vi "SubVI_ResAcc2.vi"() -> ()   [LabVIEW 2013]
uses:
  <vilib>/DAQmx/read.llb/DAQmx Read.vi
  <vilib>/DAQmx/read.llb/DAQmx Read (Analog 1D Wfm NChan NSamp).vi
  <vilib>/DAQmx/create/channels.llb/DAQmx Create Channel (TEDS-AI-Voltage-Basic).vi
  <vilib>/DAQmx/create/channels.llb/DAQmx Create Channel (AI-Voltage-Basic).vi
  <vilib>/DAQmx/configure/timing.llb/DAQmx Timing (Sample Clock).vi
  <vilib>/DAQmx/configure/trigger.llb/DAQmx Trigger.vi
  <vilib>/DAQmx/configure/trigger.llb/DAQmx Start Trigger (Digital Edge).vi
  <vilib>/DAQmx/miscellaneous.llb/DAQmx Fill In Error Info.vi
panel:
  out "task out":refnum<k21> caption="태스크 출력"
  out "error out":errorcluster caption="에러 출력"
  in  "error in":errorcluster caption="에러 입력"
  in  "timeout (s)":dbl=10.0 caption="타임아웃(초)" format="%0.2f"
  out "data":dynamicdata(graph) caption="데이터"
  in  "stop (T)":bool=TRUE caption="정지(T)"
  in  "디바이스 이름":tag="cDAQ1Mod1"
  in  "속도":dbl=100000.0
  in  "샘플 개수":i32=2000
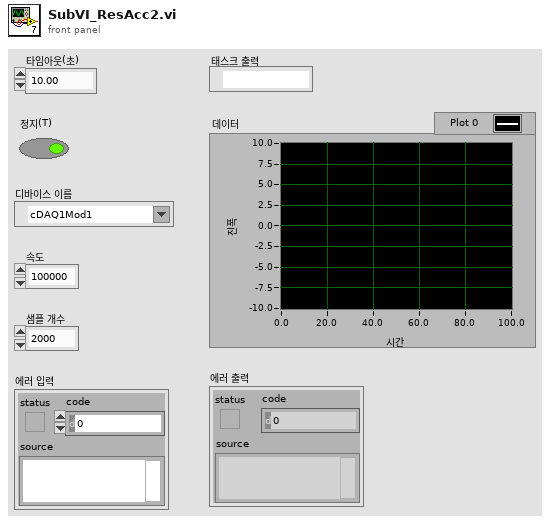
[diagram p1: front panel]
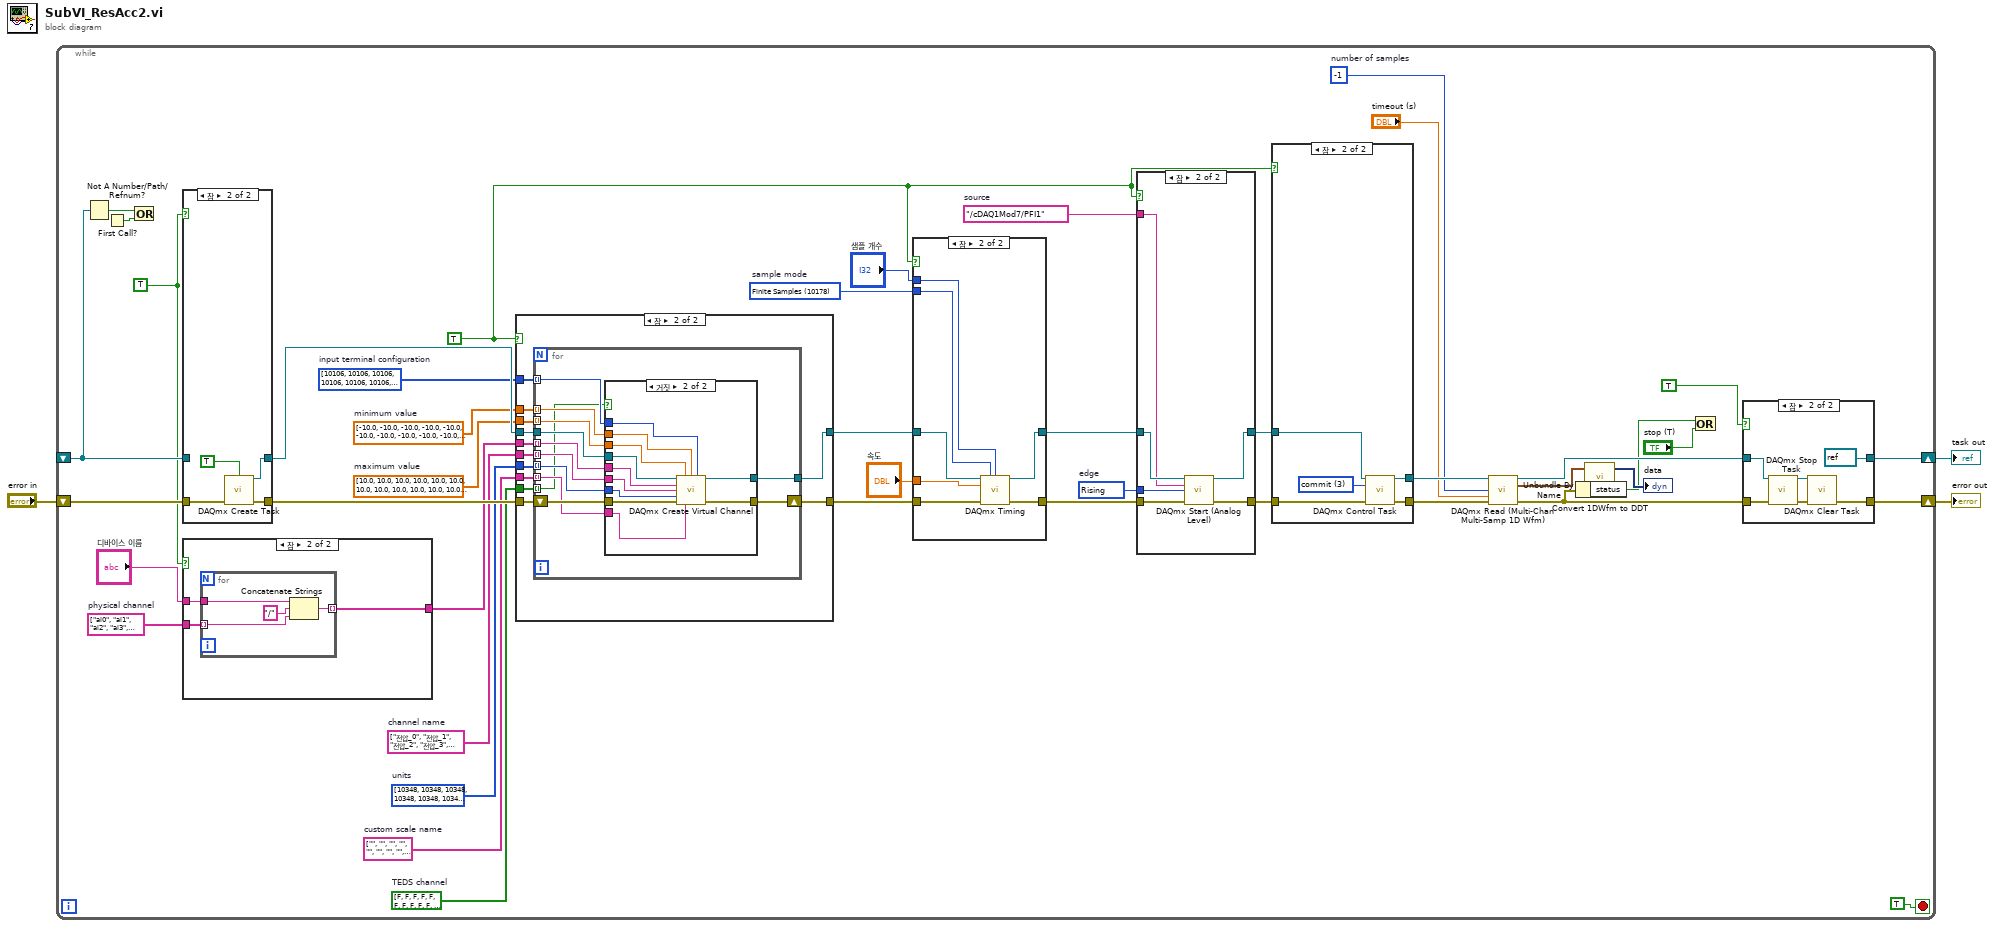
[diagram p0: block diagram]
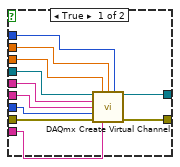
[diagram p7: hidden frame]
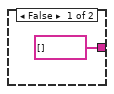
[diagram p8: hidden frame]
diagram:
  n1 = while {
    shift-right: [w12] -> w1
    shift-left: _ -> [w43]
    shift-right: [w10] -> w2
    shift-left: "error in" -> [w44]
    stop <- TRUE stop-if-true
    w5 = TRUE
    w6 = TRUE
    w16 = -1  # number of samples
    w21 = 10280 items=["Rising"=10280, "Falling"=10171]  # edge
    w22 = "/cDAQ1Mod7/PFI1"  # source
    w25 = 10178 items=["Finite Samples"=10178, "Continuous Samples"=10123, "Hardware Timed Single Point"=12522]  # sample mode
    w30 = bool[] [FALSE, FALSE, FALSE, FALSE, FALSE, FALSE, FALSE, FALSE, FALSE, FALSE, FALSE, FALSE, FALSE, FALSE, FALSE, FALSE]  # TEDS channel
    w31 = string[] ["", "", "", "", "", "", "", "", "", "", "", "", "", "", "", ""]  # custom scale name
    w32 = i32[] [10348, 10348, 10348, 10348, 10348, 10348, 10348, 10348, 10348, 10348, 10348, 10348, 10348, 10348, 10348, 10348] items=["Volts"=10348, "From TEDS"=12516, "From Custom Scale"=10065]  # units
    w33 = string[] ["전압_0", "전압_1", "전압_2", "전압_3", "전압_4", "전압_5", "전압_6", "전압_7", "전압_8", "전압_9", "전압_10", "전압_11", "전압_12", "전압_13", "전압_14", "전압_15"]  # channel name
    w35 = dbl[] [10.0, 10.0, 10.0, 10.0, 10.0, 10.0, 10.0, 10.0, 10.0, 10.0, 10.0, 10.0, 10.0, 10.0, 10.0, 10.0]  # maximum value
    w36 = dbl[] [-10.0, -10.0, -10.0, -10.0, -10.0, -10.0, -10.0, -10.0, -10.0, -10.0, -10.0, -10.0, -10.0, -10.0, -10.0, -10.0]  # minimum value
    w37 = i32[] [10106, 10106, 10106, 10106, 10106, 10106, 10106, 10106, 10106, 10106, 10106, 10106, 10106, 10106, 10106, 10106] items=["default"=-1, "RSE"=10083, "NRSE"=10078, "Differential"=10106, "Pseudodifferential"=12529]  # input terminal configuration
    w40 = string[] ["ai0", "ai1", "ai2", "ai3", "ai4", "ai5", "ai6", "ai7", "ai8", "ai9", "ai10", "ai11", "ai12", "ai13", "ai14", "ai15"]  # physical channel
    n2 = Not A Number/Path/Refnum?(number/path/refnum=w43) -> (NaN/Path/Refnum?=w42:bool)
    n3 = First Call?() -> (First Call?: T/F=w45:bool)
    n4 = Or(x=w42, y=w45) -> ()  [unwired: 1 out]
    n5 = case "케이스 구조" shown="참" w5 {
      tunnel: [w136 w140] -> w39
      tunnel: w43 -> [w136 _]
      tunnel: [w135 w139] -> w38
      tunnel: w44 -> [w135 w137]
      frame False {
      }
      frame True {
        n6 = call <vilib>:"DAQmx Create Task.vi"("auto cleanup"=TRUE, "error in"=w137) -> ("task out"=w140:refnum<k21>, "error out"=w139:errorcluster)  [unwired: 12 in]
      }
    }
    n7 = case "케이스 구조" shown="참" w5 {
      tunnel: [string[] [] w130] -> w34
      tunnel: "디바이스 이름" -> [_ w129]
      tunnel: w40 -> [_ w128]
      frame False {
      }
      frame True {
        n8 = for "For 루프" {
          tunnel: [w134] -> w130 mode=indexing
          tunnel: w129 -> [w133]
          tunnel: w128 -> [w131] mode=indexing
          n9 = Concatenate Strings(w133, "/" ("string"), w131) -> (w134:string)
        }
      }
    }
    n10 = case "케이스 구조" shown="참" w6 {
      tunnel: [w80 w90] -> w29
      tunnel: w39 -> [w80 w92]
      tunnel: [w79 w89] -> w28
      tunnel: w38 -> [w79 w91]
      tunnel: w37 -> [_ w88]
      tunnel: w36 -> [_ w87]
      tunnel: w35 -> [_ w86]
      tunnel: w34 -> [_ w85]
      tunnel: w33 -> [_ w84]
      tunnel: w32 -> [_ w83]
      tunnel: w31 -> [_ w82]
      tunnel: w30 -> [_ w81]
      frame False {
      }
      frame True {
        n11 = for "For 루프" {
          tunnel: w92 -> [w104]
          tunnel: [w102] -> w90
          tunnel: w88 -> [w100] mode=indexing
          tunnel: w87 -> [w99] mode=indexing
          tunnel: w86 -> [w98] mode=indexing
          tunnel: w85 -> [w97] mode=indexing
          tunnel: w84 -> [w96] mode=indexing
          tunnel: w83 -> [w95] mode=indexing
          tunnel: w82 -> [w94] mode=indexing
          shift-right: [w101] -> w89
          shift-left: w91 -> [w103]
          tunnel: w81 -> [w93] mode=indexing
          n12 = case "케이스 구조" shown="거짓" w93 {
            tunnel: w104 -> [w115 w126]
            tunnel: w103 -> [w114 w125]
            tunnel: [w113 w124] -> w102
            tunnel: [w112 w123] -> w101
            tunnel: w100 -> [w111 w122]
            tunnel: w99 -> [w110 w121]
            tunnel: w98 -> [w109 w120]
            tunnel: w97 -> [w108 w119]
            tunnel: w96 -> [w107 w118]
            tunnel: w95 -> [w106 w117]
            tunnel: w94 -> [w105 w116]
            frame True {
              n13 = call-poly <vilib>:"DAQmx Create Virtual Channel.vi"("task in"=w115, "maximum value"=w109, "minimum value"=w110, "input terminal configuration"=w111, "physical channels"=w108, "name to assign"=w107, "units"=w106, "error in"=w114, "custom scale name"=w105) -> ("task out"=w113:refnum<k21>, "error out"=w112:errorcluster)  [unwired: 5 in]
            }
            frame False {
              n14 = call-poly <vilib>:"DAQmx Create Virtual Channel.vi"("task in"=w126, "maximum value"=w120, "minimum value"=w121, "input terminal configuration"=w122, "physical channels"=w119, "name to assign"=w118, "units"=w117, "error in"=w125, "custom scale name"=w116) -> ("task out"=w124:refnum<k21>, "error out"=w123:errorcluster)  [unwired: 5 in]
            }
          }
        }
      }
    }
    n15 = case "케이스 구조" shown="참" w6 {
      tunnel: [w71 w73] -> w24
      tunnel: w29 -> [w71 w76]
      tunnel: [w70 w72] -> w23
      tunnel: w28 -> [w70 w74]
      tunnel: "샘플 개수" -> [_ w78]
      tunnel: w25 -> [_ w77]
      tunnel: "속도" -> [_ w75]
      frame False {
      }
      frame True {
        n16 = call-poly <vilib>:"DAQmx Timing.vi"("task/channels in"=w76, "sample mode"=w77, "samples per channel"=w78, "rate"=w75, "error in"=w74) -> ("task out"=w73:refnum<k21>, "error out"=w72:errorcluster)  [unwired: 9 in]
      }
    }
    n17 = case "케이스 구조" shown="참" w6 {
      tunnel: [w63 w67] -> w20
      tunnel: w24 -> [w63 w69]
      tunnel: [w62 w66] -> w19
      tunnel: w23 -> [w62 w68]
      tunnel: w22 -> [_ w65]
      tunnel: w21 -> [_ w64]
      frame False {
      }
      frame True {
        n18 = call-poly "DAQmx Start (Analog Level).vi"("task/channels in"=w69, "source"=w65, "edge"=w64, "error in"=w68) -> ("task out"=w67:refnum<k21>, "error out"=w66:errorcluster)  [unwired: 10 in]
      }
    }
    n19 = case "케이스 구조" shown="참" w6 {
      tunnel: [w56 w60] -> w18
      tunnel: w20 -> [w56 w61]
      tunnel: [w55 w58] -> w17
      tunnel: w19 -> [w55 w59]
      frame False {
      }
      frame True {
        w57 = 3 items=["verify"=2, "reserve"=4, "commit"=3, "unreserve"=5, "abort"=6] ("action")
        n20 = call <vilib>:"DAQmx Control Task.vi"("task/channels in"=w61, "action"=w57, "error in"=w59) -> ("task out"=w60:refnum<k21>, "error out"=w58:errorcluster)  [unwired: 11 in]
      }
    }
    n21 = call-poly "DAQmx Read (Multi-Chan Multi-Samp 1D Wfm).vi"("task/channels in"=w18, "number of samples per channel"=w16, "timeout"="timeout (s)", "error in"=w17) -> ("task out"=w11:refnum<k21>, "data"=w15:waveform(dbl)[], "error out"=w9:errorcluster)  [unwired: 9 in]
    n22 = Unbundle By Name(w9) -> ("status"=w8:bool)
    n23 = call <vilib>:"Convert 1DWfm to DDT.vi"("Array of Waveforms"=w15) -> ("Dynamic Data Type"=→"data":dynamicdata)  [unwired: 3 in]
    n24 = Or(x=w8, y="stop (T)") -> ()  [unwired: 1 out]
    n25 = case "케이스 구조" shown="참" TRUE {
      tunnel: [w48 refnum<k21> refnum ("task in")] -> w12
      tunnel: w11 -> [w48 w54]
      tunnel: [w47 w51] -> w10
      tunnel: w9 -> [w47 w53]
      frame False {
      }
      frame True {
        n26 = call <vilib>:"DAQmx Stop Task.vi"("task/channels in"=w54, "error in"=w53) -> ("task out"=w50:refnum<k21>, "error out"=w52:errorcluster)  [unwired: 12 in]
        n27 = call <vilib>:"DAQmx Clear Task.vi"("task in"=w50, "error in"=w52) -> ("error out"=w51:errorcluster)  [unwired: 13 in]
      }
    }
  }
  "error out" <- w2
  "task out" <- w1
